vi "Event Set Event (Data).vi"(8 "error in (no error)":errorcluster, 9 "Data":refnum<data-value>, 10 "Event name":string, 11 "Event DVR in":refnum<data-value>) -> (0 "error out":errorcluster, 3 "Event DVR out":refnum<data-value>)   [LabVIEW 2012, in "MDSplus.lvlib"]
doc: "Issues a new event."
uses:
  <vilib>/MDSplus/Library/MDSplus.lvlib
  <vilib>/MDSplus/Classes/Event_Class/Event.lvclass
  <vilib>/MDSplus/Classes/Data_Class/Data.lvclass
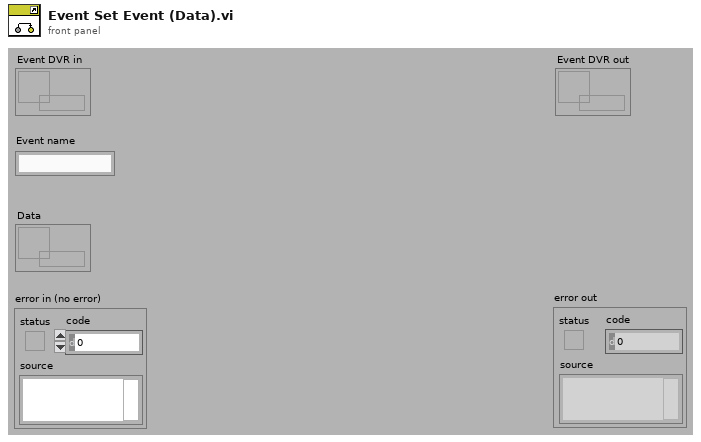
[diagram p1: front panel]
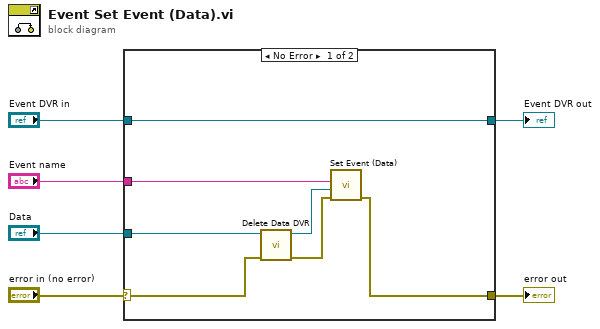
[diagram p0: block diagram]
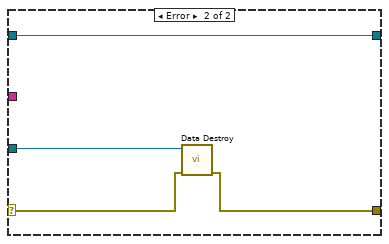
[diagram p2: hidden frame]
diagram:
  n1 = case shown="No Error" "error in (no error)" {
    selector: "error in (no error)" -> [w9 w15]
    tunnel: "Event DVR in" -> [w7 w17]
    tunnel: [w8 w14] -> w6
    tunnel: [w7 w17] -> w3
    tunnel: "Data" -> [w13 w16]
    tunnel: "Event name" -> [w12 _]
    frame No Error {
      n2 = call <vilib>:"Delete Data DVR.vi"("error in (no error)"=w9, "Data DVR in"=w13) -> ("error out"=w11:errorcluster, "Data out"=w10:refnum<class "Data.lvclass">)  [unwired: 8 in]
      n3 = call <vilib>:"Set Event (Data).vi"("error in (no error)"=w11, "Data"=w10, "Event name"=w12) -> ("error out"=w8:errorcluster)  [unwired: 7 in, 1 out]
    }
    frame Error {
      n4 = call <vilib>:"Data Destroy.vi"("error in (no error)"=w15, "Data DVR in"=w16) -> ("error out"=w14:errorcluster)  [unwired: 9 in]
    }
  }
  "error out" <- w6
  "Event DVR out" <- w3
